vi "logger_loop.vi"(8 "error in":errorcluster, 11 "Micron config":T1) -> (0 "error out":errorcluster)   [LabVIEW 2014]
uses:
  initialization/micron_config.ctl
  manipulator/squiggle/Host/i2c_interface.ctl
  manipulator/squiggle/Host/fpga_reference.ctl
  Micron params.ctl
  stimulus.ctl
  injection_point.ctl
  filtering/goal_loop_parms.ctl
  mode_conrols.ctl
  manipulator_cal.ctl
  asap/labview/testing/probe_calibration.ctl
  host/network_params.ctl
  cancellation/sq_control_params.ctl
  cancellation/decoupled_gain.ctl
  cancellation/estimation_controls.ctl
  <vilib>/Platform/TimedLoop/XDataNode/timing_clust.ctl
  <vilib>/Platform/TimedLoop/XDataNode/nitl_modes.ctl
  <vilib>/Platform/TimedLoop/XDataNode/wakeup.ctl
  probe_point.ctl
  initialization/micron_globals.vi
  <vilib>/Platform/TimedLoop/XDataNode/XDataNode.xnode
  <vilib>/Platform/TimedLoop/XDataNode/XDNodeRunTimeDep.lvlib
panel:
  out "UDP write error":errorcluster
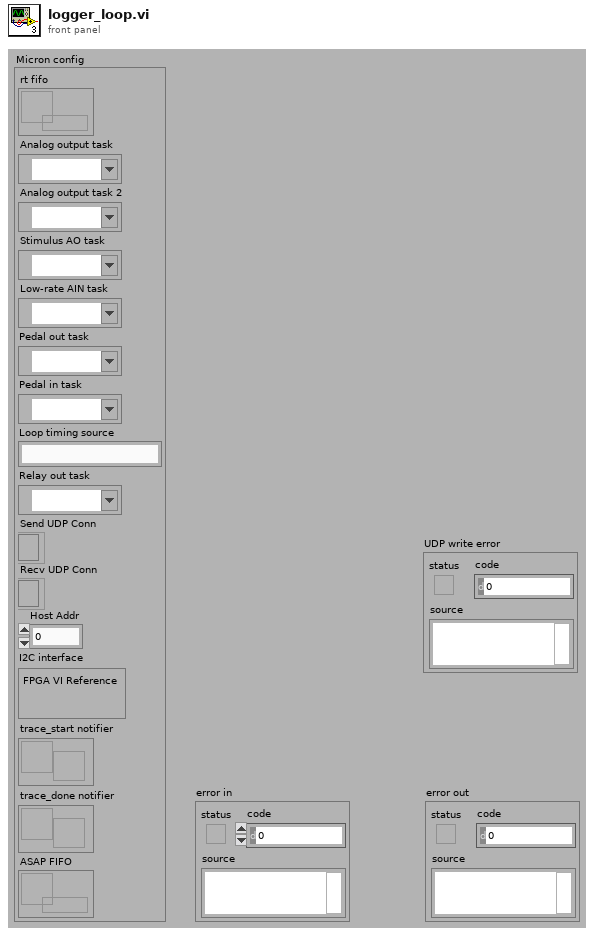
[diagram p1: front panel]
types:
  T1 = typedef "micron_config.ctl" = cluster{"rt fifo":refnum<k33>, "Analog output task":refnum<k21>, "Analog output task 2":refnum<k21>, "Stimulus AO task":refnum<k21>, "Low-rate AIN task":refnum<k21>, "Pedal out task":refnum<k21>, "Pedal in task":refnum<k21>, "Loop timing source":string, "Relay out task":refnum<k21>, "Send UDP Conn":refnum<k16>, "Recv UDP Conn":refnum<k16>, "Host Addr":u32, "I2C interface":T2, "trace_start notifier":refnum<notifier>, "trace_done notifier":refnum<notifier>, "ASAP FIFO":refnum<k33>}
  T2 = typedef "i2c_interface.ctl" = cluster{"FPGA VI Reference":T3}
  T3 = typedef "fpga_reference.ctl" = refnum<k20>
  T4 = typedef "Micron params.ctl" = cluster{"Stimulus":T5, "Goal Filter A":T7, "Mode controls":T8, "Manipulator type":enum16{"Current piezo", "Voltage piezo"}, "Manipulator calibration":T9, "Network":T11, "Goal Filter B":T7, "Cancellation":T12, "Transition time":sgl, "Estimation":T14}
  T5 = typedef "stimulus.ctl" = cluster{"Type":enum16{"Off", "Step", "Sine", "Triangle", "Arbitrary"}, "Phase":dbl, "Amplitude":sgl[], "Injection point":T6, "Closed loop":bool, "Offset":sgl[], "Tip -> world":bool, "Frequency":dbl, "Length":dbl}
  T6 = typedef "injection_point.ctl" = enum16{"Total pose", "V limiter", "Goal ", "Link position", "KF link position", "Inverse kin", "Link goal", "Link error", "Controller", "Output", "Drive", "Light"}
  T7 = typedef "goal_loop_parms.ctl" = cluster{"Speedup max":sgl, "Speedup thresh":sgl, "Speedup nonlin":sgl, "Filters":cluster{"Lower Fc":sgl, "Lower Q":sgl, "Scale factor":sgl, "Upper Fc":sgl, "Upper Q":sgl, "V limit":sgl, "V limit range":sgl}[]}
  T8 = typedef "mode_conrols.ctl" = cluster{"Hold":bool, "Cancellation":bool, "Goal filter":bool, "Trigger":bool}
  T9 = typedef "manipulator_cal.ctl" = cluster{"Tool offsets":sgl[][], "Tip light calibration":T10, "Handle light calibration":T10, "Base pivots":sgl[][], "Output pivots":sgl[][], "Length center":sgl, "Workspace height":sgl[], "Workspace diameter":sgl[], "Linearization":sgl[][], "Stack travel":sgl, "Saturation pos":sgl, "Inverse filters":cluster{"filter structure":enum32{"IIR 2nd Order", "IIR 4th Order"}, "Reverse Coefficients":dbl[], "Forward Coefficients":dbl[]}[]}
  T10 = typedef "probe_calibration.ctl" = sgl[][]
  T11 = typedef "network_params.ctl" = cluster{"Remote Host":string, "Send Status":bool, "Send Port":u16, "Recv Commands":bool, "Recv Port":u16}
  T12 = typedef "sq_control_params.ctl" = cluster{"KP":T13, "KI":sgl, "KD":T13, "Max vel":sgl, "Max acc":sgl, "Int error limit":sgl, "RCM gain":sgl, "Bypass":bool, "Degraded gain":sgl}
  T13 = typedef "decoupled_gain.ctl" = cluster{"XY":sgl, "Rxy":sgl, "Z":sgl, "Rz":sgl}
  T14 = typedef "estimation_controls.ctl" = cluster{"Link":cluster{"Measure noise":dbl[], "Process noise":dbl[], "Alt process noise":dbl[], "Alt turnoff cycles":i32, "Innovation limit":dbl[], "Residue threshold":dbl, "Enable":bool}, "Handle":cluster{"Measure noise":dbl[], "Process noise":dbl[], "State limits":dbl[], "Innovation limit":dbl[], "Prediction Lookahead":sgl, "Enable":bool}}
  T15 = typedef "XDNodeRunTimeDep.lvlib/timing_clust.ctl" = cluster{"Expected End [f-1]":u64, "Actual End [f-1]":u64, "Finished Late? [f-1]":bool, "Expected End [i-1]":u64, "Actual End [i-1]":u64, "Finished Late? [i-1]":bool, "Expected Start [i]":u64, "Actual Start [i]":u64, "Expected Start [f]":u64, "Actual Start [f]":u64, "Source Name":string, "Structure Name":string, "Period":i64, "Deadline":i64, "Offset":i64, "Start":i64, "Priority":i32, "Timeout":i32, "Mode":T16, "Wakeup Reason":T17, "Error":errorcluster, "Source Type":string, "Secondary Source Type":string, "Global End Time":u64, "Global Start Time":u64, "Frame Duration":u64, "Iteration Duration":u64, "Assigned CPU":i32, "I/O Scan Engine Mode":u32}
  T16 = typedef "XDNodeRunTimeDep.lvlib/nitl_modes.ctl" = enum32{"No Change", "Process missed periods, maintain original phase", "Discard missed periods, maintain original phase", "Process missed periods, ignore original phase", "Discard missed periods, ignore original phase"}
  T17 = typedef "XDNodeRunTimeDep.lvlib/wakeup.ctl" = enum32{"Normal", "Aborted", "Asynchronous wakeup", "Timing source error", "Timed loop error", "Timeout"}
  T18 = typedef "probe_point.ctl" = enum16{"Position (tip)", "Position (RCM)", "Null pos (tip)", "Null pos (RCM)", "V limiter (tip)", "V Limiter (RCM)", "Goal filter (tip)", "Goal filter (RCM)", "Goal force (tip)", "Goal force (RCM)", "Goal (tip)", "Goal (RCM)", "Link pos 0", "Link pos 1", "KF link pos 0", "KF link pos 1", "Link rate 0", "Link rate 1", "Link residue 0", "Link residue 1", "Link goal 0", "Link goal 1", "Rate limit 0", "Rate limit 1", "Link error 0", "Link error 1", "Controller 0", "Controller 1", "Output 0", "Output 1", "Drive 0", "Drive 1", "Stimulus 0", "Stimulus 1", "Trace data 0", "Trace data 1", "Analog data 0", "Analog data 1", "Status flags", "Light 0", "Light 1", "Light 2", "Light 3", "Light 4", "Light 5", "Goal origin", "Goal rotation 0", "Goal rotation 1", "Goal rotation 2", "Output origin", "Output rotation 0", "Output rotation 1", "Output rotation 2", "Handle origin", "Handle rotation 0", "Handle rotation 1", "Handle rotation 2", "Handle position", "Handle velocity", "Handle acceleration", "Handle angles", "Handle angle rates", "Handle pos residue", "Handle angle residue", "Trace length"}
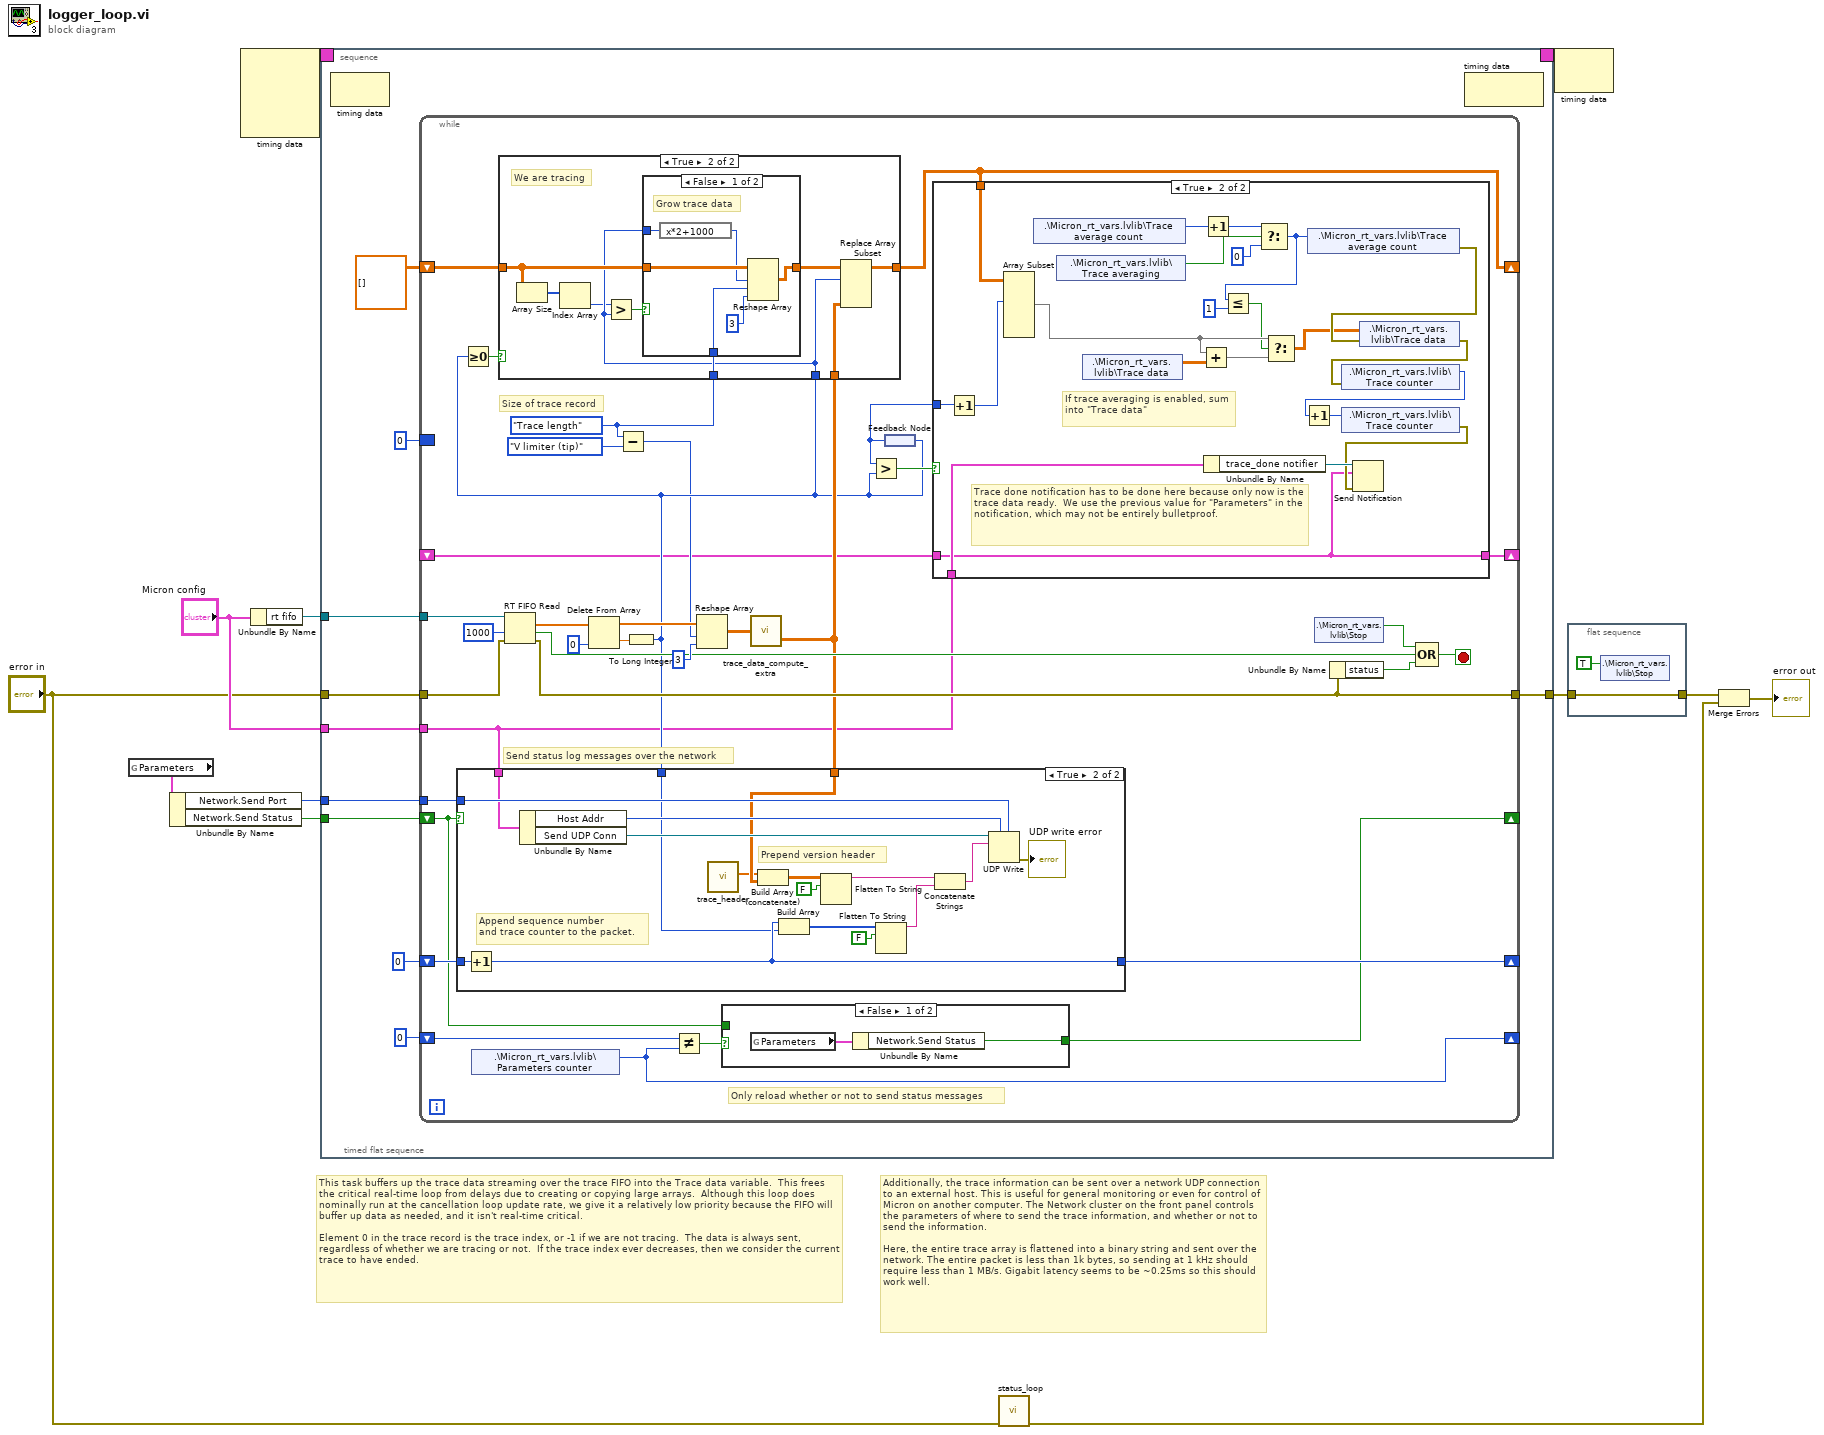
[diagram p0: block diagram]
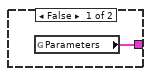
[diagram p6: hidden frame]
diagram:
  # "Additionally, the trace information can be sent over a network UDP connection to an external host. This is useful for general monitoring or even for control of Micron on another computer. The Network cluster on the front panel controls the parameters of where to send the trace information, and whether or not to send the information. \n\nHere, the entire trace array is flattened into a binary string and sent over the network. The entire packet is less than 1k bytes, so sending at 1 kHz should require less than 1 MB/s. Gigabit latency seems to be ~0.25ms so this should work well."
  # "This task buffers up the trace data streaming over the trace FIFO into the Trace data variable.  This frees the critical real-time loop from delays due to creating or copying large arrays.  Although this loop does nominally run at the cancellation loop update rate, we give it a relatively low priority because the FIFO will buffer up data as needed, and it isn't real-time critical.\n\nElement 0 in the trace record is the trace index, or -1 if we are not tracing.  The data is always sent, regardless of whether we are tracing or not.  If the trace index ever decreases, then we consider the current trace to have ended."
  n1 = global read "micron_globals.vi" "Parameters"() -> (w7:T4)
  n2 = Unbundle By Name(w7) -> ("Network.Send Port"=w9:u16, "Network.Send Status"=w8:bool)
  n3 = node-c288() -> (w12:T15)  [unwired: 1 in, 3 out]
  n4 = Unbundle By Name("Micron config") -> ("rt fifo"=w10:refnum<k33>)
  n5 = timed-sequence {
    timing: w12 -> [_]
    timing-out: [_] -> w11
    tunnel: w10 -> [w18]
    tunnel: [w17] -> w5
    tunnel: "error in" -> [w16]
    tunnel: w9 -> [w15]
    tunnel: w8 -> [w14]
    tunnel: "Micron config" -> [w13]
    n6 = timed-flat-sequence {
      tunnel: w18 -> [w27]
      tunnel: [w25] -> w17
      tunnel: w16 -> [w24]
      tunnel: w15 -> [w23]
      tunnel: w14 -> [w22]
      tunnel: w13 -> [w20]
      n7 = node-c288() -> ()  [unwired: 2 out]
      n8 = while {
        tunnel: w27 -> [w63]
        shift-right: [w58] -> _
        shift-left: sgl[][][] [] -> [w59]
        tunnel: [w50] -> w25
        tunnel: w24 -> [w49]
        border: 0 -> [_]
        tunnel: w23 -> [w47]
        shift-right: [w45] -> _
        shift-left: u32 0 -> [w46]
        shift-right: [w40] -> _
        shift-left: u32 0 ("Parameters counter") -> [w44]
        shift-right: [w41] -> _
        shift-left: w22 -> [w42]
        tunnel: w20 -> [w31]
        shift-right: [w30] -> _
        shift-left: _ -> [w29]
        stop <- w56 stop-if-true
        w34 = probe_point."Trace length" ("Injection point")
        # "Size of trace record"
        # "Send status log messages over the network"
        # "Only reload whether or not to send status messages"
        n9 = shared-variable ".\\Micron_rt_vars.lvlib\\Parameters counter"() -> (w40:u32)  [unwired: 2 out]
        n10 = RT FIFO Read(0:w63, 2:1000 ("timeout in ms (0)"), 3:w49) -> (9:w62:sgl[], 10:w52:bool, 11:w50:errorcluster)  [unwired: 1 in, 2 out]
        n11 = Delete From Array(array=w62, index=0) -> (deleted portion=w60:sgl, array with subset deleted=w39:sgl[])  [unwired: 1 in]
        n12 = Subtract(x=w34, y=probe_point."V limiter (tip)" ("Injection point")) -> (x-y=w32:u16)
        n13 = To Long Integer(number=w60) -> (32bit integer=w35:i32)
        n14 = Greater Or Equal To 0?(x=w35) -> (x >= 0?=w37:bool)
        n15 = Not Equal?(x=w44, y=w40) -> (x != y?=w43:bool)
        n16 = Reshape Array(w39, w32, 3 ("dimension size")) -> (w38:sgl[][])
        n17 = case shown="False" w43 {
          tunnel: [w81 w83] -> w41
          tunnel: w42 -> [_ w83]
          frame False {
            n18 = global read "micron_globals.vi" "Parameters"() -> (w82:T4)
            n19 = Unbundle By Name(w82) -> ("Network.Send Status"=w81:bool)
          }
          frame True {
          }
        }
        n20 = call "trace_data_compute_extra.vi"("Input Trace"=w38) -> ("Full Trace"=w36:sgl[][])  [unwired: 1 out]
        n21 = case shown="True" w42 {
          tunnel: w47 -> [_ w101]
          tunnel: w36 -> [_ w95]
          tunnel: w46 -> [w84 w100]
          tunnel: [w84 w88] -> w45
          tunnel: w31 -> [_ w96]
          tunnel: w35 -> [_ w87]
          frame False {
          }
          frame True {
            # "Prepend version header"
            # "Append sequence number\nand trace counter to the packet."
            n22 = Increment(x=w100) -> (x+1=w88:u32)
            n23 = Unbundle By Name(w96) -> ("Host Addr"=w98:u32, "Send UDP Conn"=w97:refnum<k16>)
            n24 = call "trace_header.vi"() -> ("Header"=w93:sgl[])  [unwired: 11 in]
            n25 = Build Array (concatenate)(w93, w95) -> (w99:sgl[][])
            n26 = Build Array(w88, w87) -> (w86:u32[])
            n27 = Flatten To String(anything=w99, prepend array or string size? (T)=FALSE) -> (data string=w91:string)  [unwired: 1 in, 3 out]
            n28 = Flatten To String(anything=w86, prepend array or string size? (T)=FALSE) -> (data string=w89:string)  [unwired: 1 in, 3 out]
            n29 = Concatenate Strings(w91, w89) -> (w92:string)
            n30 = UDP Write(address=w98, port or service name=w101, connection ID=w97, data in=w92) -> (error out=→"UDP write error":errorcluster)  [unwired: 1 in, 2 out]
          }
        }
        n31 = case shown="True" w37 {
          tunnel: w59 -> [w64 w68]
          tunnel: [w64 w72] -> w58
          tunnel: w34 -> [_ w71]
          tunnel: w36 -> [_ w70]
          tunnel: w35 -> [_ w66]
          frame False {
          }
          frame True {
            # "We are tracing"
            n32 = Array Size(array=w68) -> (size(s)=w69:i32[])
            n33 = Index Array(array=w69) -> (element=w65:i32)  [unwired: 1 in]
            n34 = Greater?(x=w65, y=w66) -> (0:w67:bool)
            n35 = case shown="False" w67 {
              tunnel: w68 -> [w78 w80]
              tunnel: [w74 w80] -> w73
              tunnel: w71 -> [w76 _]
              tunnel: w66 -> [w79 _]
              frame False {
                # "Grow trace data"
                n36 = expression code="x*2+1000"(w79) -> (w77:i32)
                n37 = Reshape Array(w78, w77, w76, 3 ("dimension size")) -> (w74:sgl[][][])
              }
              frame True {
              }
            }
            n38 = Replace Array Subset(array=w73, new element=w70, index (dim 0)=w66) -> (w72:sgl[][][])  [unwired: 2 in]
          }
        }
        n39 = feedback-in #1(w35) -> ()
        n40 = feedback #1() -> (w55:i32)
        n41 = Greater?(x=w55, y=w35) -> (0:w48:bool)
        n42 = case shown="True" w48 {
          tunnel: w58 -> [_ w124]
          tunnel: w55 -> [_ w123]
          tunnel: w31 -> [_ w106]
          tunnel: [w102 w103] -> w30
          tunnel: w29 -> [_ w103]
          frame False {
            n43 = global read "micron_globals.vi" "Parameters"() -> (w102:T4)
          }
          frame True {
            # "Trace done notification has to be done here because only now is the trace data ready.  We use the previous value for \"Parameters\" in the notification, which may not be entirely bulletproof."
            # "If trace averaging is enabled, sum into \"Trace data\""
            n44 = Increment(x=w123) -> (x+1=w122:i32)
            n45 = Array Subset(array=w124, length (dim 0)=w122) -> (w110:sgl[][][])  [unwired: 5 in]
            n46 = shared-variable ".\\Micron_rt_vars.lvlib\\Trace average count"() -> (w113:u32)  [unwired: 2 out]
            n47 = shared-variable ".\\Micron_rt_vars.lvlib\\Trace averaging"() -> (w116:bool)  [unwired: 2 out]
            n48 = shared-variable ".\\Micron_rt_vars.lvlib\\Trace data"() -> (w117:sgl[][][])  [unwired: 2 out]
            n49 = Add(x=w110, y=w117) -> (x+y=w111:sgl[][][])
            n50 = Increment(x=w113) -> (x+1=w115:u32)
            n51 = Unbundle By Name(w106) -> ("trace_done notifier"=w105:refnum<notifier>)
            n52 = Select(t=w115, s=w116, f=u32 0 ("x+1")) -> (s? t:f=w109:u32)
            n53 = Less Or Equal?(x=w109, y=u32 1) -> (x <= y?=w107:bool)
            n54 = Select(t=w110, s=w107, f=w111) -> (s? t:f=w112:sgl[][][])
            n55 = shared-variable ".\\Micron_rt_vars.lvlib\\Trace average count"(w109) -> (error out=w118:errorcluster)  [unwired: 1 out]
            n56 = shared-variable ".\\Micron_rt_vars.lvlib\\Trace data"(w112, error in=w118) -> (error out=w119:errorcluster)
            n57 = shared-variable ".\\Micron_rt_vars.lvlib\\Trace counter"(error in=w119) -> (w120:u32)  [unwired: 1 out]
            n58 = Increment(x=w120) -> (x+1=w121:u32)
            n59 = shared-variable ".\\Micron_rt_vars.lvlib\\Trace counter"(w121) -> (error out=w104:errorcluster)  [unwired: 1 out]
            n60 = Send Notification(notification=w103, notifier=w105, error in (no error)=w104) -> ()  [unwired: 2 out]
          }
        }
        n61 = shared-variable ".\\Micron_rt_vars.lvlib\\Stop"() -> (w53:bool)  [unwired: 2 out]
        n62 = Unbundle By Name(w50) -> ("status"=w51:bool)
        n63 = Compound Arithmetic op=OR(w53, w52, w51) -> (w56:bool)
      }
      n64 = node-c288() -> ()  [unwired: 2 out]
    }
  }
  n65 = call "status_loop.vi"("error in (no error)"="error in") -> ("error out"=w1:errorcluster)  [unwired: 10 in]
  n66 = node-c288(w11) -> ()  [unwired: 1 out]
  n67 = flat-sequence {
    tunnel: w5 -> [w127]
    tunnel: [w127] -> w3
    frame #0 {
      n68 = shared-variable ".\\Micron_rt_vars.lvlib\\Stop"(TRUE ("Stop")) -> ()  [unwired: 2 out]
    }
  }
  n69 = Merge Errors(w3, w1) -> (→"error out":errorcluster)
